vi "MoveReplicate.vi"(7 "Team Index":i32, 10 "View":i32[](array[numeric]) caption="View (Team Index, -1: empty)") -> (1 "Direction":T2, 2 "Action":T1)   [LabVIEW 2016, in "AndrewF.lvclass"]
uses:
  AndrewF.lvclass
  Type Defs/Direction Enum.ctl
  Type Defs/Action Enum.ctl
  Type Defs/SB Type Defs.lvlib
  Common/Common.lvlib
panel:
  # "NW\nN\nNE\nE\nSE\nS\nSW\nW"
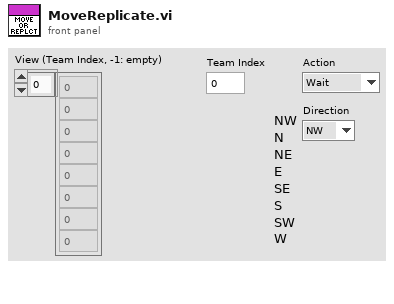
[diagram p1: front panel]
types:
  T1 = typedef "SB Type Defs.lvlib/Action Enum.ctl" = enum16{"Wait", "Move", "Attack", "Replicate"}
  T2 = typedef "SB Type Defs.lvlib/Direction Enum.ctl" = enum16{"NW", "N", "NE", "E", "SE", "S", "SW", "W"}
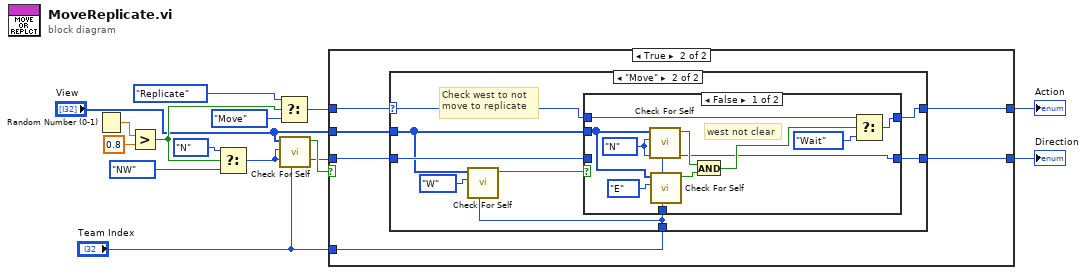
[diagram p0: block diagram]
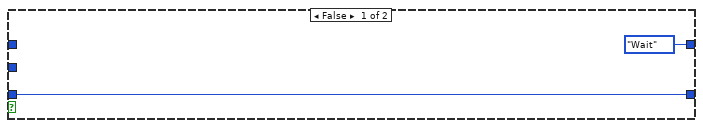
[diagram p2: hidden frame]
diagram:
  n1 = Random Number (0-1)() -> (number: 0 to 1=w14:dbl)
  n2 = Greater?(x=w14, y=0.8) -> (0:w8:bool)
  n3 = Select(t=Direction_Enum."N" ("Direction"), s=w8, f=Direction_Enum."NW") -> (s? t:f=w5:T2)
  n4 = Select(t=Action_Enum."Replicate" ("Action"), s=w8, f=Action_Enum."Move" ("Action")) -> (s? t:f=w6:T1)
  n5 = call "Check For Self.vi"("Team index"="Team Index", "Direction"=w5, "Map"="View") -> ("Clear?"=w7:bool)  [unwired: 8 in]
  n6 = case shown="True" w7 {
    tunnel: [Action_Enum."Wait" ("f") w21] -> w2
    tunnel: "View" -> [_ w22]
    tunnel: w6 -> [_ w20]
    tunnel: [w15 w18] -> w3
    tunnel: w5 -> [w15 w19]
    tunnel: "Team Index" -> [_ w17]
    frame False {
    }
    frame True {
      n7 = case shown="\"Move\"" w20 {
        selector: w20 -> [w24 w29]
        tunnel: w22 -> [_ w27]
        tunnel: [w24 w28] -> w21
        tunnel: w19 -> [w23 w31]
        tunnel: [w23 w30] -> w18
        tunnel: w17 -> [_ w25]
        frame "Wait", Default {
        }
        frame "Move" {
          # "Check west to not\nmove to replicate"
          n8 = call "Check For Self.vi"("Team index"=w25, "Direction"=Direction_Enum."W", "Map"=w27) -> ("Clear?"=w26:bool)  [unwired: 8 in]
          n9 = case shown="False" w26 {
            tunnel: w31 -> [_ w43]
            tunnel: [w34 w43] -> w30
            tunnel: w29 -> [w42 w44]
            tunnel: [w40 w44] -> w28
            tunnel: w27 -> [w38 _]
            tunnel: w25 -> [w33 _]
            frame False {
              w34 = Direction_Enum."N" ("Direction")
              # "west not clear"
              n10 = call "Check For Self.vi"("Team index"=w33, "Direction"=w34, "Map"=w38) -> ("Clear?"=w37:bool)  [unwired: 8 in]
              n11 = call "Check For Self.vi"("Team index"=w33, "Direction"=Direction_Enum."E", "Map"=w38) -> ("Clear?"=w36:bool)  [unwired: 8 in]
              n12 = And(x=w37, y=w36) -> (x .and. y?=w35:bool)
              n13 = Select(t=w42, s=w35, f=Action_Enum."Wait") -> (s? t:f=w40:T1)
            }
            frame True {
            }
          }
        }
      }
    }
  }
  "Direction" <- w3
  "Action" <- w2
